vi "模拟输入_保存_csv.vi"() -> ()   [LabVIEW 2013]
doc: "This example demonstrates how to acquire a continuous data."
uses:
  <userlib>/ArtDAQ/_SubVI/ArtDAQ_CreateAIVoltageChan.vi
  <userlib>/ArtDAQ/_SubVI/ArtDAQ_CfgSampClkTiming.vi
  <userlib>/ArtDAQ/_SubVI/ArtDAQ_CfgDigEdgeStartTrig.vi
  <userlib>/ArtDAQ/_SubVI/ArtDAQ_CfgAnlgEdgeStartTrig.vi
  <userlib>/ArtDAQ/_SubVI/ArtDAQ_CfgAnlgWindowStartTrig.vi
  <userlib>/ArtDAQ/_SubVI/ArtDAQ_Read Analog DBL NChan NSamp.vi
  <vilib>/Utility/file.llb/Write To Spreadsheet File (DBL).vi
panel:
  in  "文件路径":path=path "C:/Users/Administrator/Desktop/Data.csv"
  in  "触发模式":enum32{"无触发", "数字边沿", "模拟边沿", "模拟窗"}(tab)
  in  "触发源":string="/Dev1/PFI1"
  in  "触发边沿":i32(ring)=10280 items=["上升"=10280, "下降"=10171]
  in  "触发电平(V)":dbl
  in  "触发源":string(combo)="Dev1/ai0"
  in  "斜率":i32(ring)=10280 items=["上升"=10280, "下降"=10171]
  in  "触发条件":i32(ring)=10163 items=["进入窗"=10163, "离开窗"=10208]
  in  "窗顶部":dbl=0.5
  in  "窗底部":dbl
  in  "触发源":string(combo)="Dev1/ai0"
  in  "停止":bool
  out "Waveform":dbl[][](graph)
  in  "采样频率":dbl=10000.0 format="%#_13g"
  in  "每通道采样点数":i32=1000
  in  "接地方式":i32(ring)=10083 items=["默认"=-1, "单端"=10083, "非参考单端"=10078, "差分"=10106, "伪差分"=12529]
  in  "最小值(V)":dbl=-10.0 format="%#_13g"
  in  "最大值(V)":dbl=10.0 format="%#_13g"
  in  "物理通道":string(combo)="Dev1/ai0"
  out "错误":errorcluster
  # "通道属性"
  # "定时"
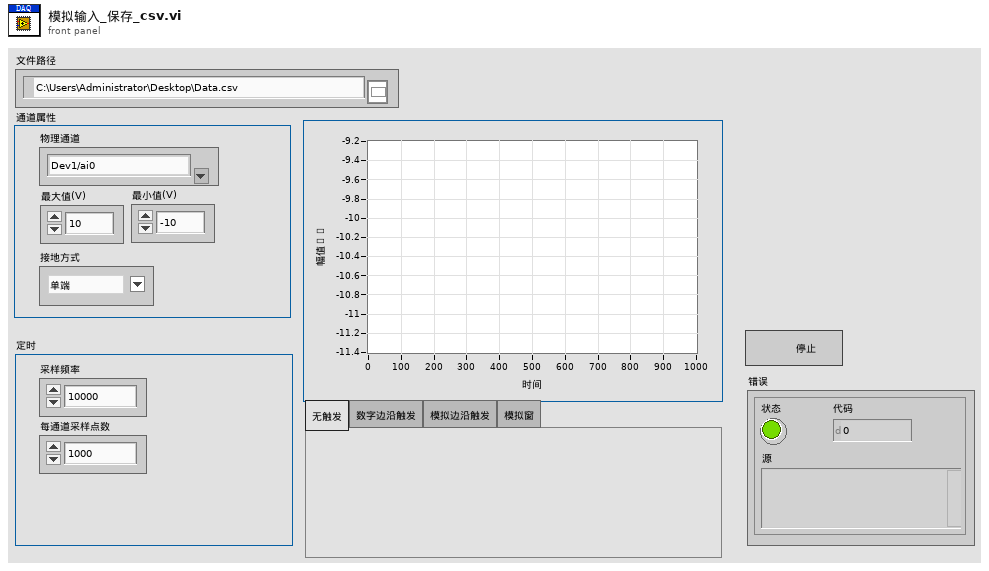
[diagram p1: front panel]
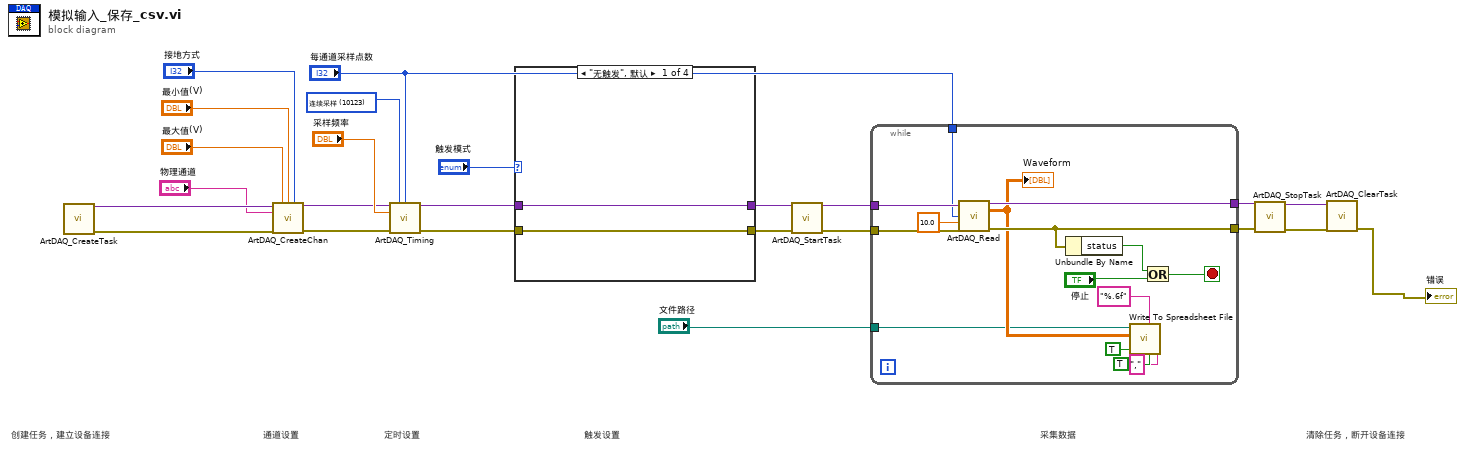
[diagram p0: block diagram]
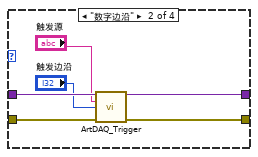
[diagram p2: hidden frame]
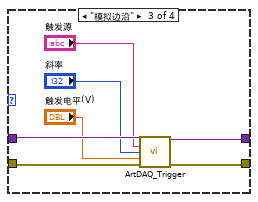
[diagram p3: hidden frame]
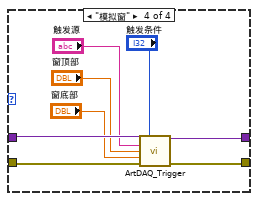
[diagram p4: hidden frame]
diagram:
  w4 = 10123 items=["有限点采样"=10178, "连续采样"=10123] ("SampleMode")
  # "清除任务，断开设备连接"
  # "采集数据"
  # "触发设置"
  # "定时设置"
  # "通道设置"
  # "创建任务，建立设备连接"
  n1 = call <userlib>:"ArtDAQ_CreateTask.vi"() -> ("任务句柄"=w15:variant, "错误输出"=w24:errorcluster)  [unwired: 14 in]
  n2 = call-poly <userlib>:"ArtDAQ_CreateChan.vi"("任务句柄"=w15, "最大值"="最大值(V)", "最小值"="最小值(V)", "接线端配置"="接地方式", "物理通道"="物理通道", "错误输入"=w24) -> ("任务句柄"=w5:variant, "错误输出"=w20:errorcluster)  [unwired: 8 in]
  n3 = call-poly <userlib>:"ArtDAQ_Timing.vi"("任务句柄"=w5, "采样模式"=w4, "每通道采样数"="每通道采样点数", "采样率"="采样频率", "错误输入"=w20) -> ("任务句柄"=w9:variant, "错误输出"=w7:errorcluster)  [unwired: 9 in]
  n4 = case shown="\"无触发\", 默认" "触发模式" {
    tunnel: w9 -> [w26 w32 w39 w47]
    tunnel: [w26 w31 w38 w46] -> w8
    tunnel: w7 -> [w25 w29 w36 w44]
    tunnel: [w25 w30 w37 w45] -> w6
    frame "无触发", Default {
    }
    frame "数字边沿" {
      n5 = call-poly <userlib>:"ArtDAQ_Trigger.vi"("任务句柄"=w32, "触发源"="触发源", "边沿"="触发边沿", "错误输入"=w29) -> ("任务句柄"=w31:variant, "错误输出"=w30:errorcluster)  [unwired: 10 in]
    }
    frame "模拟边沿" {
      n6 = call-poly <userlib>:"ArtDAQ_Trigger.vi"("任务句柄"=w39, "触发源"="触发源", "斜率"="斜率", "触发电平"="触发电平(V)", "错误输入"=w36) -> ("任务句柄"=w38:variant, "错误输出"=w37:errorcluster)  [unwired: 9 in]
    }
    frame "模拟窗" {
      n7 = call-poly <userlib>:"ArtDAQ_Trigger.vi"("任务句柄"=w47, "触发条件"="触发条件", "触发源"="触发源", "窗顶部"="窗顶部", "窗底部"="窗底部", "错误输入"=w44) -> ("任务句柄"=w46:variant, "错误输出"=w45:errorcluster)  [unwired: 8 in]
    }
  }
  n8 = call <userlib>:"ArtDAQ_StartTask.vi"("任务句柄"=w8, "错误输入"=w6) -> ("任务句柄"=w18:variant, "错误输出"=w17:errorcluster)  [unwired: 12 in]
  n9 = while {
    tunnel: w18 -> [w62]
    tunnel: w17 -> [w61]
    tunnel: "每通道采样点数" -> [w60]
    tunnel: [w58] -> w14
    tunnel: [w57] -> w13
    tunnel: "文件路径" -> [w49]
    stop <- w55 stop-if-true
    n10 = call-poly <userlib>:"ArtDAQ_Read.vi"("任务句柄"=w62, "每通道采样数"=w60, "超时s"=10.0 ("Timeout"), "错误输入"=w61) -> ("任务句柄"=w58:variant, "数据"=w53:dbl[][], "错误输出"=w57:errorcluster)  [unwired: 8 in, 1 out]
    "Waveform" <- w53
    n11 = Unbundle By Name(w57) -> ("status"=w56:bool)
    n12 = call-poly <vilib>:"Write To Spreadsheet File.vi"("delimiter (\\t)"="," ("delimiter (\\t)"), "transpose? (no:F)"=TRUE, "format (%.3f)"="%.6f", "append to file? (new file:F)"=TRUE, "2D data"=w53, "file path (dialog if empty)"=w49) -> ()  [unwired: 2 in, 1 out]
    n13 = Or(x=w56, y="停止") -> (x .or. y?=w55:bool)
  }
  n14 = call <userlib>:"ArtDAQ_StopTask.vi"("任务句柄"=w14, "错误输入"=w13) -> ("任务句柄"=w12:variant, "错误输出"=w11:errorcluster)  [unwired: 12 in]
  n15 = call <userlib>:"ArtDAQ_ClearTask.vi"("任务句柄"=w12, "错误输入"=w11) -> ("错误输出"=→"错误":errorcluster)  [unwired: 13 in]
